vi "FLA.vi"(0 "System no.":i32=1 min=1 step=1, 1 "Board":i32=1 min=1 max=5 step=1, 2 "Axis to scan":string, 3 "Decrease VEL\nfor scan?":bool, 4 "Range":dbl=0.1 format="%.4f", 5 "error in":errorcluster, 6 "Treshold level":dbl=0.1 format="%.3f", 7 "Step size":dbl=0.001 format="%.4f", 8 "AA step size":dbl=0.0001 format="%.4f", 9 "Velocity":dbl=0.2 format="%.4f", 10 "Use #7 polling?":bool, 11 "Timeout (s)":dbl=300.0 min=1.0 max=4.0 step=1.0 format="%.2f", 12 "Stop refnum":refnum<vi>) -> (14 "Scan successful?":bool, 19 "error out":errorcluster)   [LabVIEW 2026]
doc: "Performs a line scan and align in specified axis, waits until scan is ready using #7 polling and indicates whether scan was successful or not. If Refnum stop or Local stop is TRUE, VI sends #24 and stops."
uses:
  Communication/Syntax.ctl
  Communication/Global1.vi
panel:
  in  "Local stop":bool
  # "Performs a line scan and align in specified axis, waits until scan is ready\nusing #7 polling and indicates whether scan was successful or not. If \nStop refnum or Local stop is TRUE, VI sends #24 and stops."
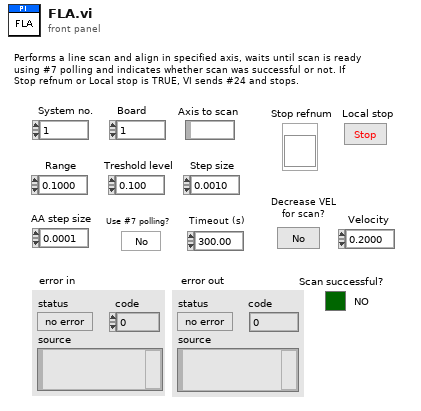
[diagram p1: front panel]
types:
  T1 = typedef "Syntax.ctl" = enum16{"GCS 1.0", "GCS 2.0", "GCS 3.0"}
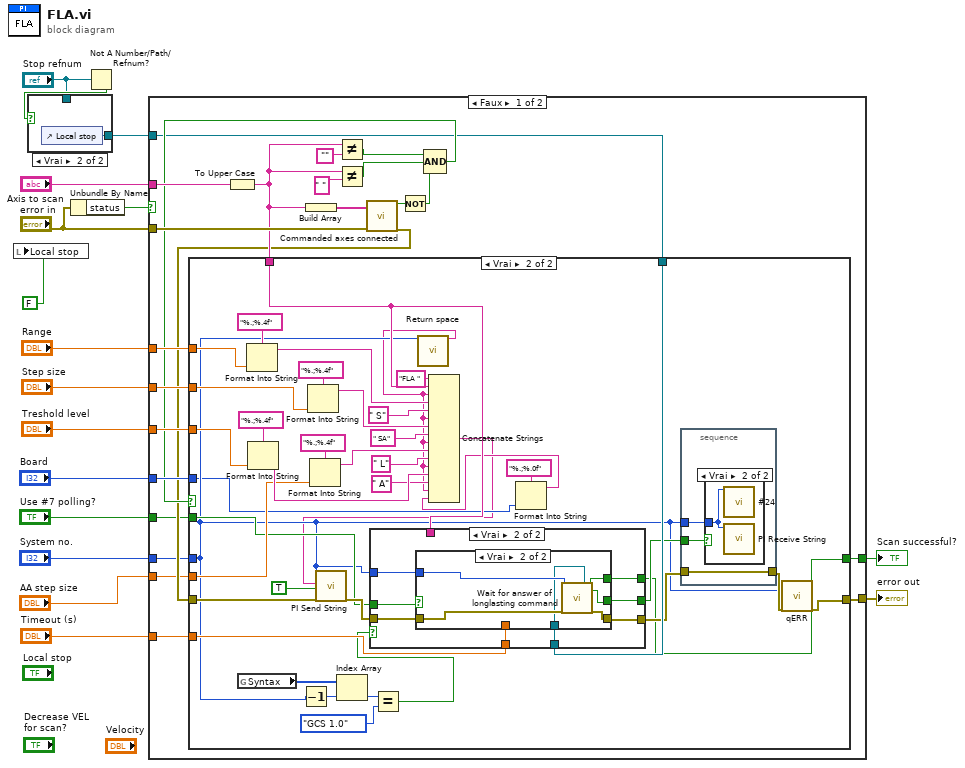
[diagram p0: block diagram]
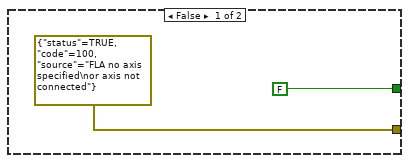
[diagram p3: hidden frame]
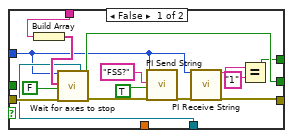
[diagram p4: hidden frame]
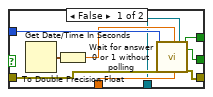
[diagram p5: hidden frame]
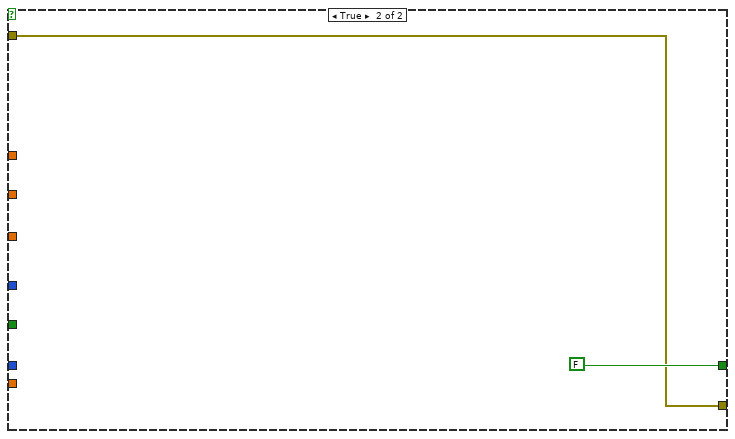
[diagram p7: hidden frame]
diagram:
  n1 = local write "Local stop"(FALSE ("Local stop")) -> ()
  n2 = Unbundle By Name("error in") -> ("status"=w12:bool)
  n3 = Not A Number/Path/Refnum?(number/path/refnum="Stop refnum") -> (NaN/Path/Refnum?=w5:bool)
  n4 = case shown="Vrai" w5 {
    tunnel: [w18 w19] -> w3
    tunnel: "Stop refnum" -> [w18 _]
    frame False {
    }
    frame True {
      n5 = control-ref of="Local stop"() -> (w19:refnum<vi>)
    }
  }
  n6 = case shown="Faux" w12 {
    tunnel: "System no." -> [w28 _]
    tunnel: [w27 w127] -> w16
    tunnel: "Axis to scan" -> [w42 _]
    tunnel: [w26 FALSE] -> w14
    tunnel: "error in" -> [w36 w127]
    tunnel: "Board" -> [w35 _]
    tunnel: "Range" -> [w34 _]
    tunnel: "Step size" -> [w33 _]
    tunnel: "Treshold level" -> [w31 _]
    tunnel: "AA step size" -> [w23 _]
    tunnel: w3 -> [w22 _]
    tunnel: "Use #7 polling?" -> [w21 _]
    tunnel: "Timeout (s)" -> [w20 _]
    frame False {
      n7 = To Upper Case(1:w42) -> (0:w32:string)
      n8 = Build Array(w32) -> (w37:string[])
      n9 = Not Equal?(x=w32, y="") -> (x != y?=w39:bool)
      n10 = Not Equal?(x=w32, y=" ") -> (x != y?=w38:bool)
      n11 = call "Commanded axes connected.vi"("Commanded axes"=w37, "error in"=w36) -> ("Controller error"=w25:bool, "error out"=w29:errorcluster)  [unwired: 1 in, 15 out]
      n12 = Not(x=w25) -> (.not. x?=w24:bool)
      n13 = Compound Arithmetic op=AND(w39, w38, w24) -> (w30:bool)
      n14 = case shown="Vrai" w30 {
        tunnel: w35 -> [_ w48]
        tunnel: w34 -> [_ w80]
        tunnel: w33 -> [_ w75]
        tunnel: w32 -> [_ w62]
        tunnel: w31 -> [_ w77]
        tunnel: w29 -> [_ w83]
        tunnel: w28 -> [_ w53]
        tunnel: [errorcluster {"status"=TRUE, "code"=100, "source"="FLA no axis specified\nor axis not connected"} ("error out") w67] -> w27
        tunnel: [FALSE w58] -> w26
        tunnel: w23 -> [_ w68]
        tunnel: w22 -> [_ w61]
        tunnel: w21 -> [_ w63]
        tunnel: w20 -> [_ w57]
        frame False {
        }
        frame True {
          n15 = global read "Global1.vi" "Syntax"() -> (w54:T1[])
          n16 = Format Into String(format string="%.;%.4f" ("Format String"), w80) -> (resulting string=w79:string)  [unwired: 2 in, 1 out]
          n17 = Format Into String(format string="%.;%.4f" ("Format String"), w77) -> (resulting string=w73:string)  [unwired: 2 in, 1 out]
          n18 = Decrement(x=w53) -> (x-1=w55:i32)
          n19 = Format Into String(format string="%.;%.4f" ("Format String"), w75) -> (resulting string=w74:string)  [unwired: 2 in, 1 out]
          n20 = Format Into String(format string="%.;%.4f" ("Format String"), w68) -> (resulting string=w69:string)  [unwired: 2 in, 1 out]
          n21 = Index Array(array=w54, index=w55) -> (element=w56:T1)
          n22 = Equal?(x=w56, y=Syntax."GCS 1.0") -> (x = y?=w52:bool)
          n23 = call "Return space.vi"("System no."=w53) -> ("String out"=w50:string)  [unwired: 1 in, 17 out]
          n24 = Format Into String(format string="%.;%.0f" ("Format String"), w48) -> (resulting string=w47:string)  [unwired: 2 in, 1 out]
          n25 = Concatenate Strings("FLA ", w62, w50, w79, " S", w50, w74, " SA", w50, w69, " L", w50, w73, " A" ("Substring"), w50, w47) -> (w46:string)
          n26 = call "PI Send String.vi"("System no."=w53, "String to send"=w46, "Attach termination char.?"=TRUE ("Attach Linefeed?"), "error in"=w83) -> ("error out"=w64:errorcluster)  [unwired: 15 out]
          n27 = case shown="Vrai" w52 {
            tunnel: w63 -> [_ w107]
            tunnel: w57 -> [_ w106]
            tunnel: [w88 w105] -> w60
            tunnel: [w85 w104] -> w58
            tunnel: w61 -> [w95 w103]
            tunnel: [w94 w102] -> w59
            tunnel: w53 -> [w89 w101]
            tunnel: w64 -> [w98 w100]
            tunnel: w62 -> [w96 _]
            frame False {
              n28 = Build Array(w96) -> (w97:string[])
              n29 = call "Wait for axes to stop.vi"("System no."=w89, "Axes to wait for"=w97, "With status bit polling?"=FALSE, "error in"=w98, "Stop refnum"=w95) -> ("Stopped"=w94:bool, "error out"=w91:errorcluster)  [unwired: 2 in, 11 out]
              n30 = call "PI Send String.vi"("System no."=w89, "String to send"="FSS?", "Attach termination char.?"=TRUE ("Attach Linefeed?"), "error in"=w91) -> ("error out"=w90:errorcluster)  [unwired: 15 out]
              n31 = call "PI Receive String.vi"("System no."=w89, "error in"=w90) -> ("String read"=w86:string, "error out"=w88:errorcluster)  [unwired: 1 in, 15 out]
              n32 = Equal?(x=w86, y="1") -> (x = y?=w85:bool)
            }
            frame True {
              n33 = case shown="Vrai" w107 {
                tunnel: w101 -> [w116 w122]
                tunnel: w100 -> [w115 w121]
                tunnel: [w114 w120] -> w105
                tunnel: [w113 w119] -> w104
                tunnel: w106 -> [w111 _]
                tunnel: w103 -> [w110 w118]
                tunnel: [w109 w117] -> w102
                frame False {
                  n34 = Get Date/Time In Seconds() -> (seconds since 1Jan1904=w108:timestamp)
                  n35 = To Double Precision Float(number=w108) -> (double precision float=w112:dbl)
                  n36 = call "Wait for answer 0 or 1 without polling.vi"("System no."=w116, "error in"=w115, "Start time"=w112, "Timeout (s)"=w111, "Stop refnum"=w110) -> ("Scan successful?"=w113:bool, "Stopped"=w109:bool, "error out"=w114:errorcluster)  [unwired: 12 out]
                }
                frame True {
                  n37 = call "Wait for answer of longlasting command.vi"("System no."=w122, "error in"=w121, "Stop refnum"=w118) -> ("Answer"=w119:bool, "Stopped"=w117:bool, "error out"=w120:errorcluster)  [unwired: 14 out]
                }
              }
            }
          }
          n38 = stacked-sequence {
            tunnel: w53 -> [w125]
            tunnel: [w124] -> w66
            tunnel: w60 -> [w124]
            tunnel: w59 -> [w123]
            frame #0 {
              n39 = case shown="Vrai" w123 {
                tunnel: w125 -> [_ w126]
                frame False {
                }
                frame True {
                  n40 = call "#24.vi"("System no."=w126) -> ()  [unwired: 1 in, 18 out]
                  n41 = call "PI Receive String.vi"("System no."=w126) -> ()  [unwired: 2 in, 17 out]
                }
              }
            }
          }
          n42 = call "qERR.vi"("System no."=w53, "error in"=w66) -> ("error out"=w67:errorcluster)  [unwired: 17 out]
        }
      }
    }
    frame True {
    }
  }
  "error out" <- w16
  "Scan successful?" <- w14
